vi "Connections Panel 6.vi"(0 "Enable":bool=TRUE, 5 "error in (no error)":errorcluster) -> (13 "Input Name 10":bool caption="Input Name 5", 14 "Input Name 6":bool caption="Input Name 1", 15 "Input Name 7":bool caption="Input Name 2", 16 "Input Name 8":bool caption="Input Name 3", 17 "Input Name 9":bool caption="Input Name 4", 18 "OK":bool, 19 "error out":errorcluster)   [LabVIEW 2014]
doc: "Displays a standard dialog box that prompts users to enter information, such as a user name and password.\n--------------------\n\nThis Express VI is configured as follows:\n\nMessage to Display to the User:נא לבצע פעולות הבאות\nThe inputs are:"
panel:
  out "Input Name 12":bool caption="Input Name 5"
  in  "Input Name 11":bool caption="שדש"
  in  "Input Name 5":bool caption="שדש"
  in  "Input Name 4":bool caption="שדש"
  in  "Input Name 3":bool caption="שדש"
  in  "Input Name 2":bool caption="שדש"
  in  "Input Name 1":bool caption="עח"
  out "String":string="נא לבצע פעולות הבאות"
  in  "Cancel":bool
  in  "OK2":bool
  in  "OK1":bool
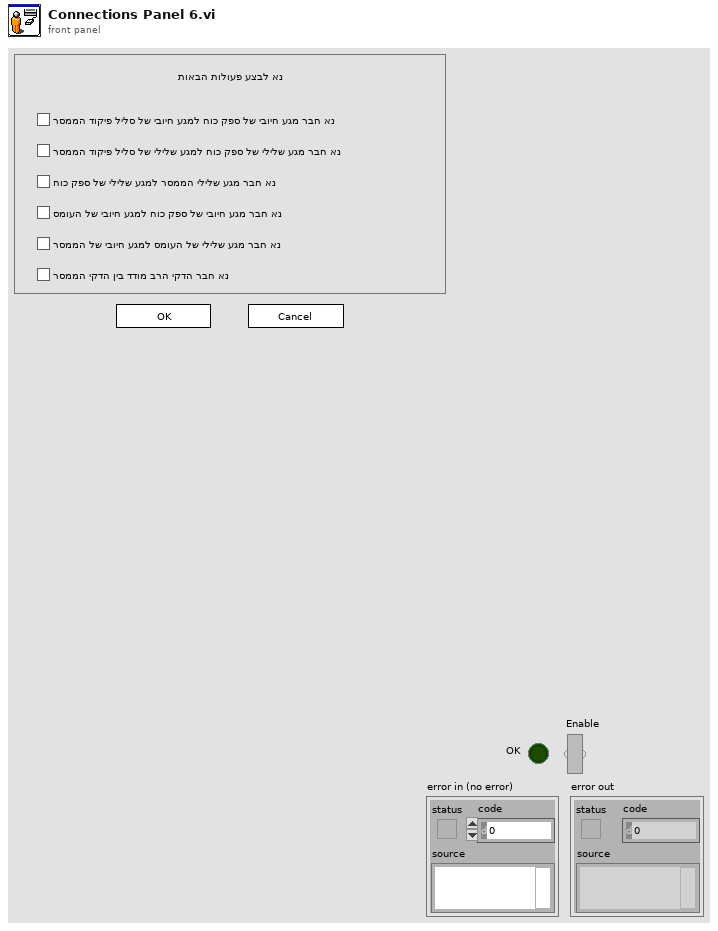
[diagram p1: front panel]
types:
  T1 = cluster{"Input Name":string, "Input Data Type":i32}[]
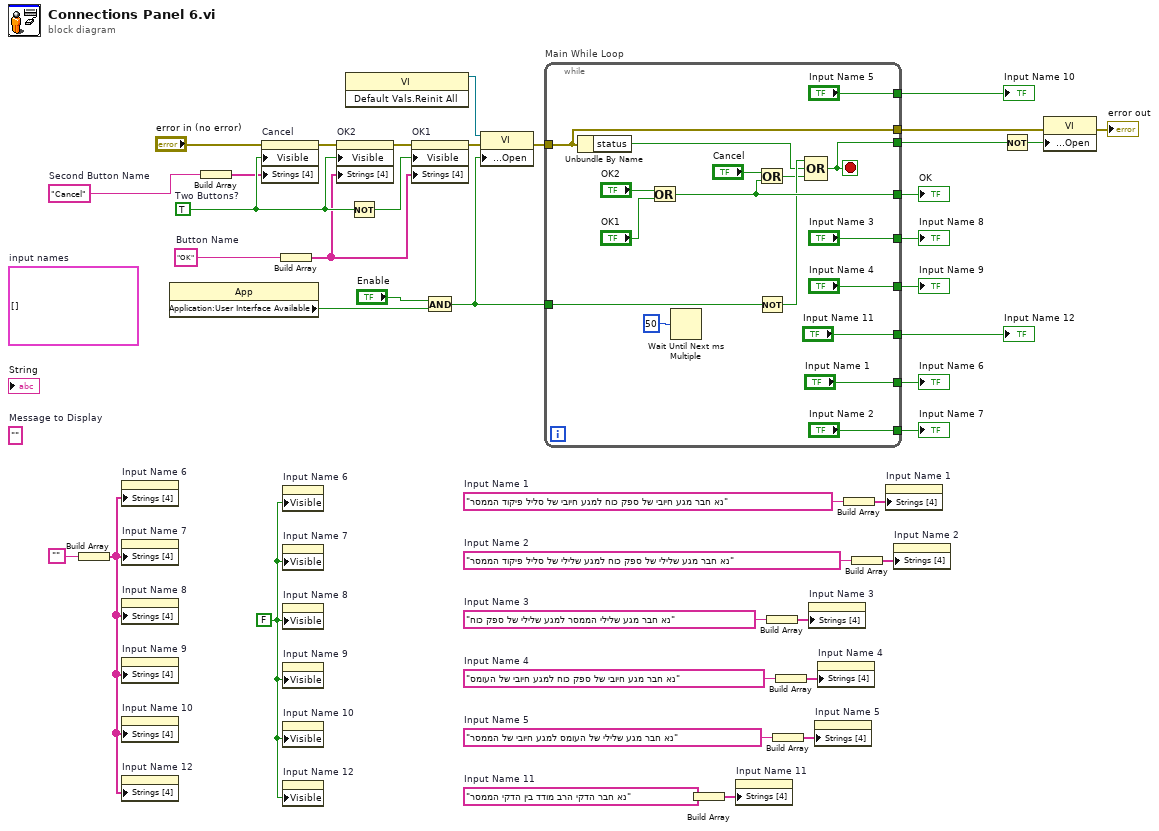
[diagram p0: block diagram]
diagram:
  w4 = "נא חבר הדקי הרב מודד בין הדקי הממסר"  # Input Name 11
  w2 = FALSE
  w10 = "נא חבר מגע שלילי של העומס למגע חיובי של הממסר"  # Input Name 5
  w11 = "נא חבר מגע חיובי של ספק כוח למגע חיובי של העומס"  # Input Name 4
  w12 = "נא חבר מגע שלילי הממסר למגע שלילי של ספק כוח"  # Input Name 3
  w15 = "נא חבר מגע שלילי של ספק כוח למגע שלילי של סליל פיקוד הממסר"  # Input Name 2
  w16 = "נא חבר מגע חיובי של ספק כוח למגע חיובי של סליל פיקוד הממסר"  # Input Name 1
  (unwired) T1 []  # input names
  w33 = "Cancel"  # Second Button Name
  w31 = "OK"  # Button Name
  (unwired) ""  # Message to Display
  w41 = TRUE  # Two Buttons?
  n1 = Build Array("") -> (w1:string[])
  n2 = property on="Input Name 6" class="Bool (strict)"("Strings [4]"=w1) -> ()  [unwired: 2 in, 2 out]
  n3 = property on="Input Name 7" class="Bool (strict)"("Strings [4]"=w1) -> ()  [unwired: 2 in, 2 out]
  n4 = property on="Input Name 8" class="Bool (strict)"("Strings [4]"=w1) -> ()  [unwired: 2 in, 2 out]
  n5 = property on="Input Name 9" class="Bool (strict)"("Strings [4]"=w1) -> ()  [unwired: 2 in, 2 out]
  n6 = property on="Input Name 10" class="Bool (strict)"("Strings [4]"=w1) -> ()  [unwired: 2 in, 2 out]
  n7 = property on="Input Name 12" class="Bool (strict)"("Strings [4]"=w1) -> ()  [unwired: 2 in, 2 out]
  n8 = property class="App"() -> ("Application:User Interface Available"=w23:bool)  [unwired: 2 in, 2 out]
  n9 = Build Array(w33) -> (w34:string[])
  n10 = property on="Cancel" class="Bool"(error in="error in (no error)", "Visible"=w41, "Strings [4]"=w34) -> (error out=w38:errorcluster)  [unwired: 1 in, 1 out]
  n11 = Build Array(w31) -> (w32:string[])
  n12 = property on="Input Name 6" class="Bool (strict)"("Visible"=w2) -> ()  [unwired: 2 in, 2 out]
  n13 = property on="Input Name 7" class="Bool (strict)"("Visible"=w2) -> ()  [unwired: 2 in, 2 out]
  n14 = property on="Input Name 8" class="Bool (strict)"("Visible"=w2) -> ()  [unwired: 2 in, 2 out]
  n15 = property on="Input Name 9" class="Bool (strict)"("Visible"=w2) -> ()  [unwired: 2 in, 2 out]
  n16 = property on="Input Name 10" class="Bool (strict)"("Visible"=w2) -> ()  [unwired: 2 in, 2 out]
  n17 = property on="Input Name 12" class="Bool (strict)"("Visible"=w2) -> ()  [unwired: 2 in, 2 out]
  n18 = property on="OK2" class="Bool"(error in=w38, "Visible"=w41, "Strings [4]"=w32) -> (error out=w37:errorcluster)  [unwired: 1 in, 1 out]
  n19 = invoke class="VI" method="Default Vals.Reinit All"() -> (reference out=w22:refnum<vi>)  [unwired: 3 in, 2 out]
  n20 = Not(x=w41) -> (.not. x?=w39:bool)
  n21 = property on="OK1" class="Bool"(error in=w37, "Visible"=w39, "Strings [4]"=w32) -> (error out=w30:errorcluster)  [unwired: 1 in, 1 out]
  n22 = And(x="Enable", y=w23) -> (x .and. y?=w24:bool)
  n23 = property class="VI"(reference=w22, error in=w30, "Front Panel Window:Open"=w24) -> (error out=w29:errorcluster)  [unwired: 1 out]
  n24 = while "Main While Loop" {
    tunnel: [w55] -> w40
    tunnel: w24 -> [w53]
    tunnel: [w51] -> w35
    tunnel: w29 -> [w50]
    tunnel: [w50] -> w27
    tunnel: ["Input Name 1"] -> w21
    tunnel: ["Input Name 2"] -> w20
    tunnel: ["Input Name 3"] -> w19
    tunnel: ["Input Name 4"] -> w18
    tunnel: ["Input Name 5"] -> w17
    tunnel: ["Input Name 11"] -> w3
    stop <- w51 stop-if-true
    n25 = Unbundle By Name(w50) -> ("status"=w48:bool)
    n26 = Or(x="OK2", y="OK1") -> (x .or. y?=w55:bool)
    n27 = Wait Until Next ms Multiple(millisecond multiple=u32 50) -> ()  [unwired: 1 out]
    n28 = Or(x="Cancel", y=w55) -> (x .or. y?=w49:bool)
    n29 = Not(x=w53) -> (.not. x?=w52:bool)
    n30 = Compound Arithmetic op=OR(w52, w48, w49) -> (w51:bool)
  }
  "OK" <- w40
  "Input Name 6" <- w21
  "Input Name 7" <- w20
  "Input Name 8" <- w19
  "Input Name 9" <- w18
  "Input Name 10" <- w17
  "Input Name 12" <- w3
  n31 = Build Array(w4) -> (w5:string[])
  n32 = property on="Input Name 11" class="Bool (strict)"("Strings [4]"=w5) -> ()  [unwired: 2 in, 2 out]
  n33 = Build Array(w12) -> (w9:string[])
  n34 = Build Array(w10) -> (w7:string[])
  n35 = Build Array(w11) -> (w8:string[])
  n36 = property on="Input Name 3" class="Bool (strict)"("Strings [4]"=w9) -> ()  [unwired: 2 in, 2 out]
  n37 = property on="Input Name 5" class="Bool (strict)"("Strings [4]"=w7) -> ()  [unwired: 2 in, 2 out]
  n38 = property on="Input Name 4" class="Bool (strict)"("Strings [4]"=w8) -> ()  [unwired: 2 in, 2 out]
  n39 = Build Array(w16) -> (w14:string[])
  n40 = Build Array(w15) -> (w13:string[])
  n41 = property on="Input Name 1" class="Bool (strict)"("Strings [4]"=w14) -> ()  [unwired: 2 in, 2 out]
  n42 = property on="Input Name 2" class="Bool (strict)"("Strings [4]"=w13) -> ()  [unwired: 2 in, 2 out]
  n43 = Not(x=w35) -> (.not. x?=w36:bool)
  n44 = property class="VI"(error in=w27, "Front Panel Window:Open"=w36) -> (error out=→"error out":errorcluster)  [unwired: 1 in, 1 out]
